vi "GetSettings.vi"(8 "error in (no error)":errorcluster, 10 "SettingsToRetrieve":variant, 11 "NHRGridSim in":refnum<class "NHRGridSim.lvclass">) -> (0 "error out":errorcluster, 2 "RetrievedSettings":variant, 3 "NHRGridSim Out":refnum<class "NHRGridSim.lvclass">)   [LabVIEW 2018, in "AcPwrPlugins.lvlib" / "NHRGridSim.lvclass"]
doc: "This VI retrieves a boolean status to see if the instrument can conduct measurements while the device is changing modes or turning off and on."
uses:
  NHRGridSim.lvclass
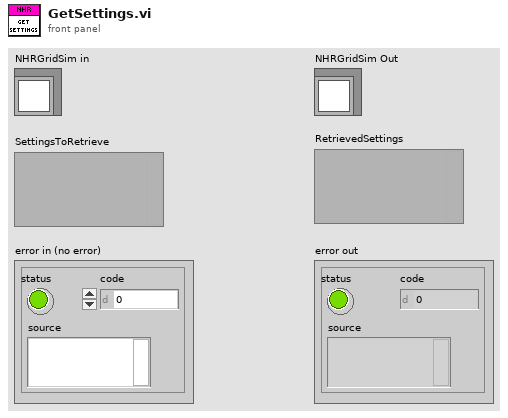
[diagram p1: front panel]
types:
  T1 = typedef "AcPwrPlugins.lvlib/NHRGridSim.lvclass/Device(s)Settings.ctl" = cluster{"MeasName":string, "Modules":T2}
  T2 = typedef "AcPwrPlugins.lvlib/NHRGridSim.lvclass/Modules.ctl" = cluster{"Measurement":cluster{"ApertureLength (s)":dbl, "NumberOfSamples":u32}, "Ranges":cluster{"Irange (A)":dbl, "Vrange (V)":dbl}, "Mode":u8, "Handle":string, "FreqOut (Hz)":dbl, "Connected":bool, "btnIdQuery":bool, "btnReset":bool, "Initialize Timeout ( ms)":u32, "Phase (0: All)":i32, "WatchDog":cluster{"Enable WatchDog":bool, "Robust WatchDog":bool, "Watchdog Interval (s)":dbl}, "Safety Limits":cluster{"Min Voltage (V)":dbl, "Min Voltage Time (s)":dbl, "Max Voltage (V)":dbl, "MaxVoltage Time (s)":dbl, "Max Source Amps (A)":dbl, "Max Source Amps Time (s)":dbl, "Max Sink Amps (A)":dbl, "Max Sink Amps Time (s)":dbl, "Max Source Power (W)":dbl, "Max Source Power Time (s)":dbl, "Max Sink Power (W)":dbl, "Max Sink Power Time (s)":dbl, "Peak Voltage (V)":dbl, "Peak Voltage Enable":bool, "Peak Amps (A)":dbl, "Peak Amps Enable":bool}, "Phases":cluster{"Pout (W)":dbl, "Iout (A)":dbl, "PhaseAngle":dbl, "Vout (V)":dbl, "Phase Name":string}[], "Regulation Gain":dbl, "ChangeOntheFly":bool, "Synchronize Output \nto Phase":bool, "Slew Rate":cluster{"Voltage Slew (Volts/s)":dbl, "Phase Angle (Degrees/s)":dbl}}[]
  T3 = cluster{"xml string":string, "xml string":string}
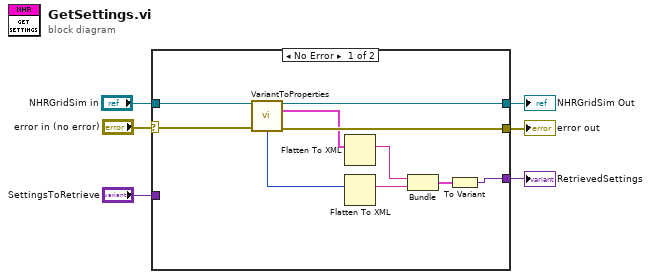
[diagram p0: block diagram]
diagram:
  n1 = case shown="No Error" "error in (no error)" {
    selector: "error in (no error)" -> [w15 w18]
    tunnel: "NHRGridSim in" -> [w16 w19]
    tunnel: [w14 w19] -> w5
    tunnel: [w13 w18] -> w1
    tunnel: "SettingsToRetrieve" -> [_ w17]
    tunnel: [w7 w17] -> w2
    frame No Error {
      n2 = call "VariantToProperties.vi"("NHRGridSim in"=w16, "error in (no error)"=w15) -> ("NHRGridSim out"=w14:refnum<class "NHRGridSim.lvclass">, "Device(s)Settings"=w8:T1, "Measurement Refresh Time (ms)"=w9:u32, "error out"=w13:errorcluster)  [unwired: 7 in, 3 out]
      n3 = Flatten To XML(anything=w8) -> (xml string=w11:string)
      n4 = Flatten To XML(anything=w9) -> (xml string=w10:string)
      n5 = Bundle("xml string"=w11, "xml string"=w10) -> (w12:T3)  [unwired: 1 in]
      n6 = To Variant(anything=w12) -> (Variant=w7:variant)
    }
    frame Error {
    }
  }
  "error out" <- w1
  "NHRGridSim Out" <- w5
  "RetrievedSettings" <- w2
